vi "Check Cluster.vi"(8 "error in":errorcluster, 11 "State":T1) -> (0 "error out":errorcluster, 3 "State out":T1)   [LabVIEW 2013]
doc: "This VI check for valid cluster names and non duplicate names"
uses:
  <vilib>/NI/DCAF/Tag Editor Core/control module/script/Controls/StateCluster.ctl
  <vilib>/NI/DCAF/Tag Editor Core/control module/script/Controls/initialized references.ctl
  <vilib>/NI/DCAF/Tag Editor Core/control module/script/Controls/interface VI type.ctl
  <vilib>/NI/DCAF/Tag Editor Core/control module/script/control module data interface generator.lvlib
panel:
  out "Elements Names":string[](array[string])
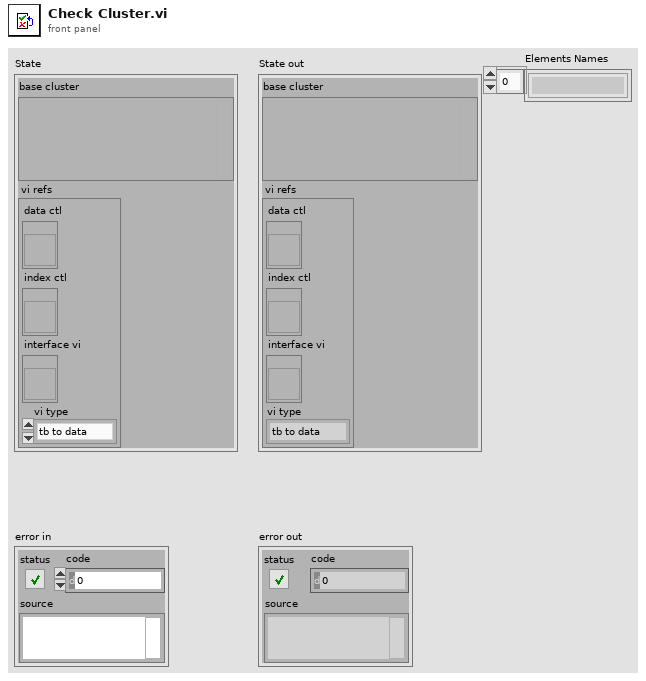
[diagram p1: front panel]
types:
  T1 = typedef "control module data interface generator.lvlib/StateCluster.ctl" = cluster{"base cluster":variant, "vi refs":T2}
  T2 = typedef "control module data interface generator.lvlib/initialized references.ctl" = cluster{"data ctl":refnum<vi>, "index ctl":refnum<vi>, "interface vi":refnum<vi>, "vi type":T3}
  T3 = typedef "control module data interface generator.lvlib/interface VI type.ctl" = enum16{"tb to data", "data to tb"}
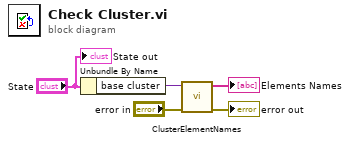
[diagram p0: block diagram]
diagram:
  n1 = Unbundle By Name("State") -> ("base cluster"=w5:variant)
  n2 = call <vilib>:"ClusterElementNames.vi"("error in"="error in", "input cluster"=w5) -> ("error out"=→"error out":errorcluster, "Elements Names"=→"Elements Names":string[])  [unwired: 5 in, 3 out]
  "State out" <- "State"
